vi "Write Sequence Version.vi"(8 "error in (no error)":errorcluster, 10 "Sequence Version":string, 11 "SequenceRepo in":refnum<class "SequenceRepo.lvclass">) -> (0 "error out":errorcluster, 3 "SequenceRepo out":refnum<class "SequenceRepo.lvclass">)   [LabVIEW 2015, in "SequenceRepo.lvclass"]
uses:
  SequenceRepo.lvclass
  SequenceRepo.lvclass/SequenceRepo.ctl
  Prototype/classes/Sequence/Config/Sequence Config.lvclass
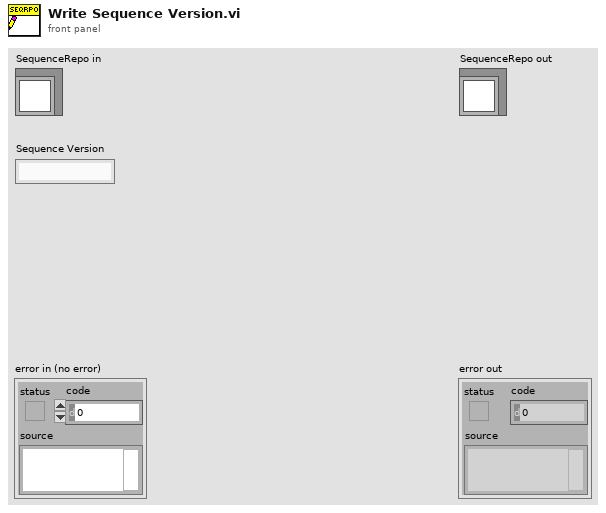
[diagram p1: front panel]
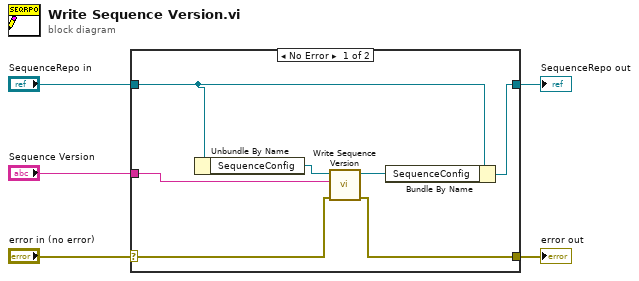
[diagram p0: block diagram]
diagram:
  n1 = case shown="No Error" "error in (no error)" {
    selector: "error in (no error)" -> [w9 w13]
    tunnel: [w10 w13] -> w4
    tunnel: [w12 w14] -> w2
    tunnel: "SequenceRepo in" -> [w7 w14]
    tunnel: "Sequence Version" -> [w8 _]
    frame No Error {
      n2 = Unbundle By Name(w7) -> ("SequenceConfig"=w6:refnum<class "Sequence Config.lvclass">)
      n3 = call-dynamic "Write Sequence Version.vi"("error in (no error)"=w9, "Sequence Version"=w8, "Sequence Config in"=w6) -> ("error out"=w10:errorcluster, "Sequence Config out"=w11:refnum<class "Sequence Config.lvclass">)  [unwired: 7 in]
      n4 = Bundle By Name(cluster=w7, "SequenceConfig"=w11) -> (w12:refnum<class "SequenceRepo.lvclass">)
    }
    frame Error {
    }
  }
  "error out" <- w4
  "SequenceRepo out" <- w2
